vi "FileAccessRead.vi"(7 "handle":u64, 8 "error in (no error)":errorcluster caption="错误输入（无错误）", 9 "pstFileAccess In":T1, 10 "pDevFileName In":i8[](array[numeric]), 11 "pUserFileName In":i8[](array[numeric])) -> (0 "error out":errorcluster caption="错误输出", 1 "pstFileAccess Out":T1, 3 "function return":i32, 5 "handle out":u64)   [LabVIEW 2015, in "MvCameraControl.lvlib"]
doc: "MV_LV_API int __stdcall SaveImage(MV_SAVE_IMAGE_PARAM* pSaveParam);"
uses:
  MvCameraControl.lvlib
  x86/MvCameraPatch.dll
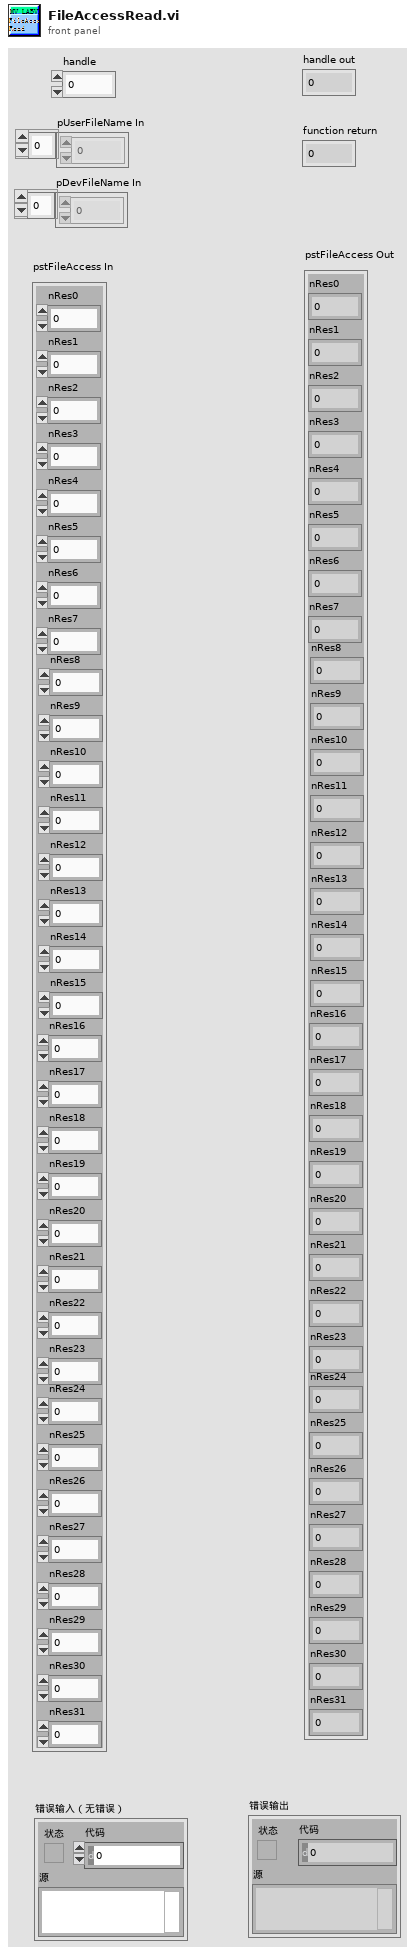
[diagram p1: front panel]
types:
  T1 = cluster{"nRes0":u32, "nRes1":u32, "nRes2":u32, "nRes3":u32, "nRes7":u32, "nRes6":u32, "nRes5":u32, "nRes4":u32, "nRes11":u32, "nRes10":u32, "nRes9":u32, "nRes8":u32, "nRes15":u32, "nRes14":u32, "nRes13":u32, "nRes12":u32, "nRes19":u32, "nRes18":u32, "nRes17":u32, "nRes16":u32, "nRes23":u32, "nRes22":u32, "nRes21":u32, "nRes20":u32, "nRes27":u32, "nRes26":u32, "nRes25":u32, "nRes24":u32, "nRes31":u32, "nRes30":u32, "nRes29":u32, "nRes28":u32}
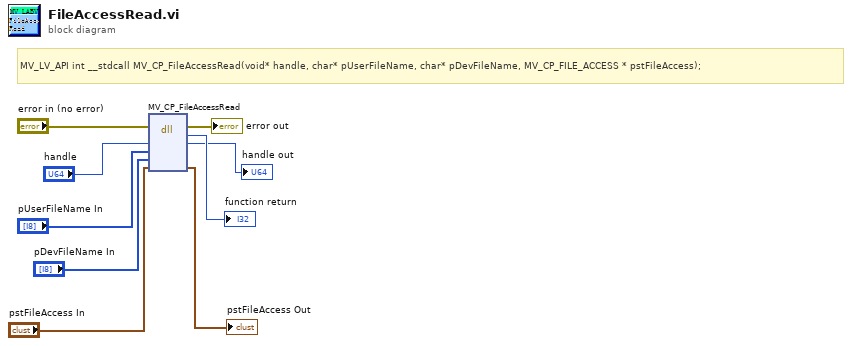
[diagram p0: block diagram]
diagram:
  # "MV_LV_API int __stdcall MV_CP_FileAccessRead(void* handle, char* pUserFileName, char* pDevFileName, MV_CP_FILE_ACCESS * pstFileAccess);"
  n1 = dll-call lib="F:/SVN/SDK/Release/MVS/Samples/Labview/MvLVLib/x86/MvCameraPatch.dll" fn="MV_CP_FileAccessRead"(error in="error in (no error)", "handle"="handle", "pUserFileName"="pUserFileName In", "pDevFileName"="pDevFileName In", "pstFileAccess"="pstFileAccess In") -> (error out=→"error out":errorcluster, "返回类型"=→"function return":i32, "handle"=→"handle out":u64, "pstFileAccess"=→"pstFileAccess Out":T1)  [unwired: 4 in, 1 out]
